vi "Assert False.vi"(6 "error code (1)":i32=1, 7 "message":string, 8 "error in (no error)":errorcluster, 11 "False?":bool) -> (0 "error out":errorcluster)   [LabVIEW 2009]
uses:
  lvlib/Pink Elephant/Pink Elephant.lvlib
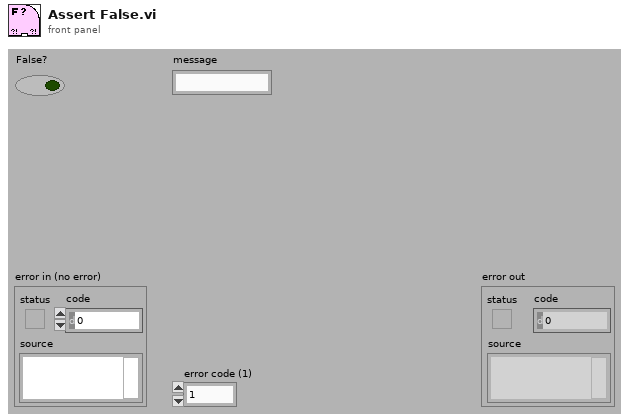
[diagram p1: front panel]
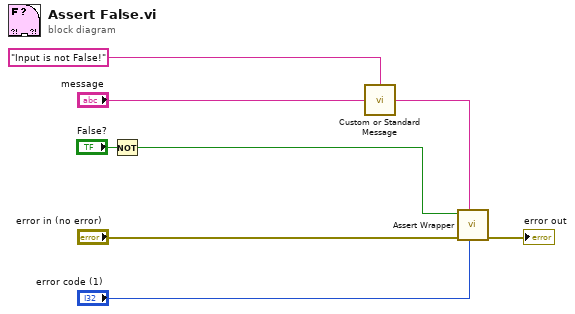
[diagram p0: block diagram]
diagram:
  n1 = Not(x="False?") -> (.not. x?=w1:bool)
  n2 = call "Custom or Standard Message.vi"("Custom Message"="message", "Standard Message"="Input is not False!") -> ("Message"=w4:string)
  n3 = call "Assert Wrapper.vi"("error code (1)"="error code (1)", "Message"=w4, "error in (no error)"="error in (no error)", "Assert?"=w1) -> ("error out"=→"error out":errorcluster)  [unwired: 7 in]
